vi "lab session 2.2V.vi"(1 "Numeric":dbl) -> (0 "Numeric 2":dbl)   [LabVIEW 2020]
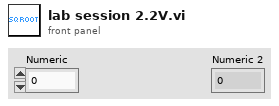
[diagram p1: front panel]
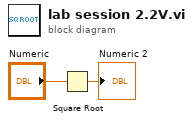
[diagram p0: block diagram]
diagram:
  n1 = Square Root(x="Numeric") -> (sqrt(x)=→"Numeric 2":dbl)
